vi "Configure Signal Path.vi"(7 "RF Converter (RX1)":i32(ring) items=["RX1", "RX2", "RX3", "RX4", "RX11", "RX12", "RX13", "RX14", "RX21", "RX22", "RX23", "RX24", "RX31", "RX32", "RX33", "RX34", "RX41", "RX42", "RX43", "RX44"], 8 "error in (no error)":errorcluster, 9 "RX Connector (RF1COM)":i32(ring) items=["RF1COM", "RF2COM", "RF3COM", "RF4COM", "R11C", "R12C", "R13C", "R14C", "R21C", "R22C", "R23C", "R24C", "R31C", "R32C", "R33C", "R34C", "R41C", "R42C", "R43C", "R44C"], 10 "Instance (1)":T1=1, 11 "VISA resource name":refnum<visa-resource-name>) -> (0 "error out":errorcluster, 3 "VISA resource name out":refnum<visa-resource-name>)   [LabVIEW 2020, in "Rohde&Schwarz CMWXP NR FR1 Measurement.lvlib"]
doc: "Selects the signal path for the measured signal.\nValue combinations:\nRF 1 COM and RF 2 COM are compatible with TX 1 and TX 3.RF 3 COM and RF 4 COM are compatible with TX 2 and TX 4.\nNote: This command is an interim solution. It is planned to replace this command in a later software version.\n\nAttribute:\nRSCMWXPNRFR1M_ATTR_SIGNAL_PATH\n\nRemote-control command:\nROUTe:NRSub:MEAS<i>:SCENario:SALone"
uses:
  <instrlib>/Rohde&Schwarz CMWXP NR FR1 Measurement/Rohde&Schwarz CMWXP NR FR1 Measurement.lvlib
  <instrlib>/Rohde&Schwarz CMWXP NR FR1 Measurement/Private/_Instance.ctl
  <instrlib>/Rohde&Schwarz CMWXP NR FR1 Measurement/Private/rsidr_core.llb/rsidr_core.lvlib
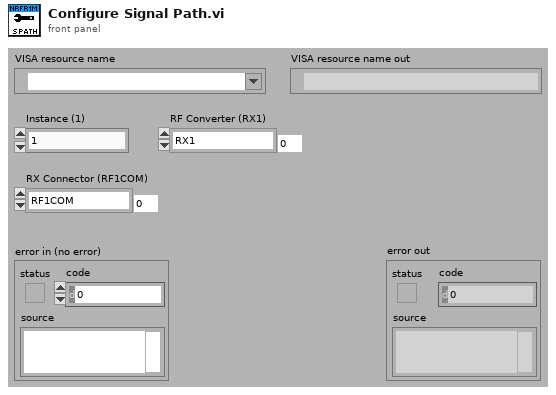
[diagram p1: front panel]
types:
  T1 = typedef "Rohde&Schwarz CMWXP NR FR1 Measurement.lvlib/_Instance.ctl" = i32
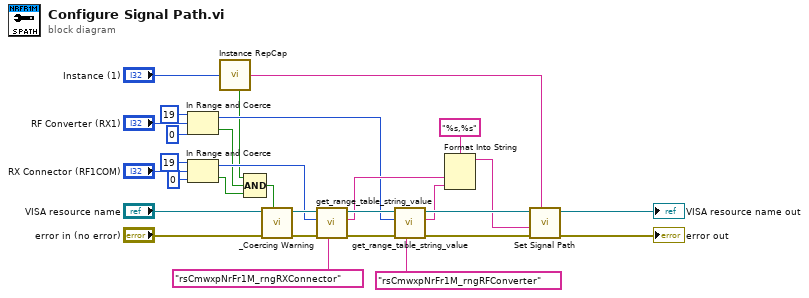
[diagram p0: block diagram]
diagram:
  n1 = In Range and Coerce(upper limit=19, x="RF Converter (RX1)", lower limit=0) -> (coerced(x)=w11:i32, In Range?=w1:bool)
  n2 = In Range and Coerce(upper limit=19, x="RX Connector (RF1COM)", lower limit=0) -> (coerced(x)=w9:i32, In Range?=w2:bool)
  n3 = call <instrlib>:"Instance RepCap.vi"("Instance In"="Instance (1)") -> ("In Range?"=w3:bool, "RepCap Identifier Out"=w26:string)  [unwired: 1 in]
  n4 = Compound Arithmetic op=AND(w3, w1, w2) -> (w4:bool)
  n5 = call <instrlib>:"_Coercing Warning.vi"("In Range?"=w4, "error in (no error)"="error in (no error)", "VISA resource name"="VISA resource name") -> ("error out"=w14:errorcluster, "VISA resource name out"=w13:refnum<visa-resource-name>)  [unwired: 7 in]
  n6 = call <instrlib>:"get_range_table_string_value.vi"("Range Table ID in"="rsCmwxpNrFr1M_rngRXConnector", "error in"=w14, "I32 input"=w9, "VISA resource name"=w13) -> ("error out"=w25:errorcluster, "String Value out"=w19:string, "VISA resource name out"=w24:refnum<visa-resource-name>)  [unwired: 5 in]
  n7 = call <instrlib>:"get_range_table_string_value.vi"("Range Table ID in"="rsCmwxpNrFr1M_rngRFConverter", "error in"=w25, "I32 input"=w11, "VISA resource name"=w24) -> ("error out"=w23:errorcluster, "String Value out"=w18:string, "VISA resource name out"=w28:refnum<visa-resource-name>)  [unwired: 5 in]
  n8 = Format Into String(format string="%s,%s", w19, w18) -> (resulting string=w17:string)  [unwired: 2 in, 1 out]
  n9 = call "Set Signal Path"("Repeated Capabilities"=w26, "error in (no error)"=w23, "Signal Path ()"=w17, "instrument handle"=w28) -> ("error out"=→"error out":errorcluster, "instrument handle out"=→"VISA resource name out":refnum<visa-resource-name>)  [unwired: 6 in]
